vi "dapo2.vi"() -> ()   [LabVIEW 2020]
panel:
  out "LOW":bool
  out "MEDIUM":bool
  out "HIGH":bool
  in  "TEMPERATURE":dbl(slide) scale=0.0..150.0
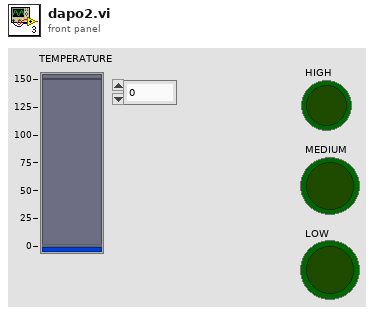
[diagram p1: front panel]
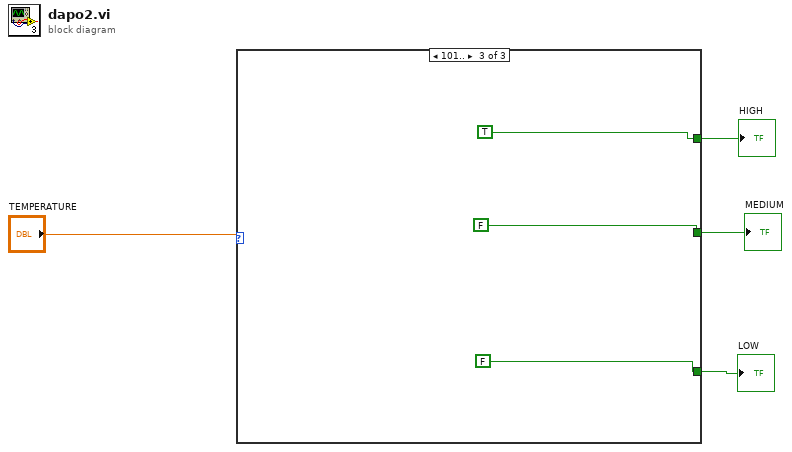
[diagram p0: block diagram]
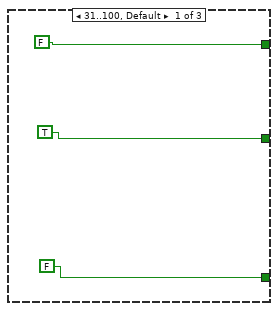
[diagram p2: hidden frame]
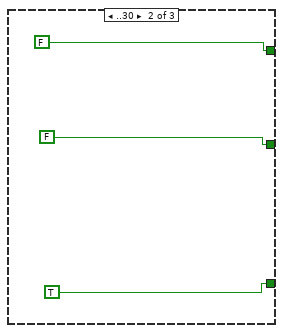
[diagram p3: hidden frame]
diagram:
  n1 = case shown="101.." "TEMPERATURE" {
    tunnel: [FALSE TRUE FALSE] -> w4
    tunnel: [TRUE FALSE FALSE] -> w3
    tunnel: [FALSE FALSE TRUE] -> w2
    frame 31..100, Default {
    }
    frame ..30 {
    }
    frame 101.. {
    }
  }
  "HIGH" <- w2
  "MEDIUM" <- w3
  "LOW" <- w4
